vi "Copy Overlay Settings.vi"(8 "error in (no error)":errorcluster, 10 "Source":refnum<class "Analyze Results Base.lvclass">, 11 "Destination":refnum<class "Analyze Results Base.lvclass">) -> (0 "error out":errorcluster, 3 "Analyze Results Base out":refnum<class "Analyze Results Base.lvclass">)   [LabVIEW 2014]
uses:
  Analyze Results Base.lvclass
  Analyze Results Base.lvclass/Analyze Results Base.ctl
  Read Overlay colors.vi
  Read Font, Size & Style.vi
  Read Overlay_.vi
  Write Overlay colors.vi
  Write Font, Size & Style.vi
  Write Overlay_.vi
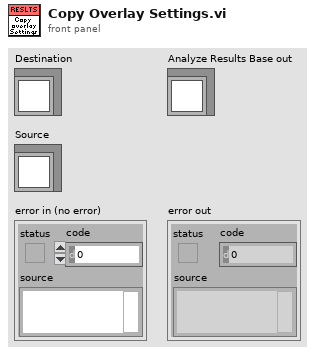
[diagram p1: front panel]
types:
  T1 = cluster{"Desired Font (Application)":enum16{"User-specified Font", "Application Font", "System Font", "Dialog Font"}, "[User-specified Font]":cluster{"Font Name":string, "Size":i16, "Strikeout?":bool, "Italic?":bool, "Underline?":bool, "Outline?":bool, "Shadow?":bool, "Bold?":bool, "Rotation Angle":dbl}, "Horizontal Alignment":i16, "Vertical Alignment":i16}
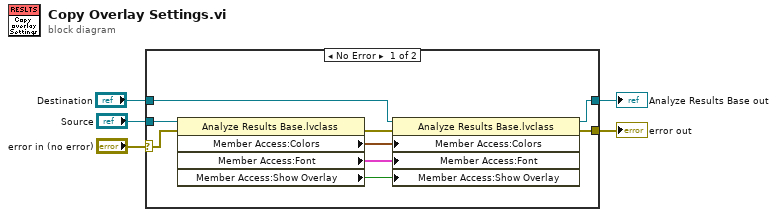
[diagram p0: block diagram]
diagram:
  n1 = case shown="No Error" "error in (no error)" {
    selector: "error in (no error)" -> [w11 w16]
    tunnel: [w6 w16] -> w4
    tunnel: [w13 w15] -> w2
    tunnel: "Destination" -> [w14 w15]
    tunnel: "Source" -> [w12 _]
    frame No Error {
      n2 = property class="Analyze Results Base.lvclass"(reference=w12, error in=w11) -> (error out=w10:errorcluster, "Member Access:Colors"=w9:cluster{"Border":u32, "Text":u32}, "Member Access:Font"=w8:T1, "Member Access:Show Overlay"=w7:bool)  [unwired: 1 out]
      n3 = property class="Analyze Results Base.lvclass"(reference=w14, error in=w10, "Member Access:Colors"=w9, "Member Access:Font"=w8, "Member Access:Show Overlay"=w7) -> (reference out=w13:refnum<class "Analyze Results Base.lvclass">, error out=w6:errorcluster)
    }
    frame Error {
    }
  }
  "error out" <- w4
  "Analyze Results Base out" <- w2
